vi "lv_factorial.vi"(9 "n":i32) -> (4 "status code":i32, 6 "out_result":i64)   [LabVIEW 2026]
uses:
  vision_core_c/bin/math_formulas.dll
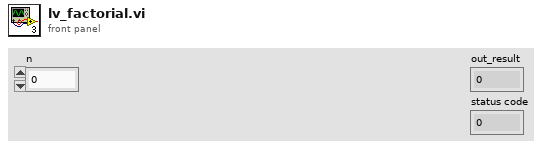
[diagram p1: front panel]
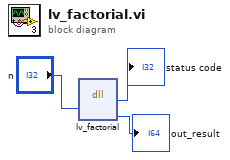
[diagram p0: block diagram]
diagram:
  n1 = dll-call lib="D:/git_proj/LabC-Vision/vision_core_c/bin/math_formulas.dll" fn="lv_factorial"("n"="n") -> ("return type"=→"status code":i32, "out_result"=→"out_result":i64)  [unwired: 5 in, 2 out]
